vi "create_file_name_discharge (SubVI).vi"(6 "file_idx":i32, 8 "num files":i32, 9 "Electrode settings:":T1={"Electrode to sweep:"=3, "amplitude (V)"=2.0, "frequency (Hz)"=41.0, "offset (V)"=0.0, "Sweep electrode?"=TRUE, "Control DDS"=TRUE}, 10 "base name":string, 11 "base_path":path) -> (2 "output cluster":T2)   [LabVIEW 2022 SP3]
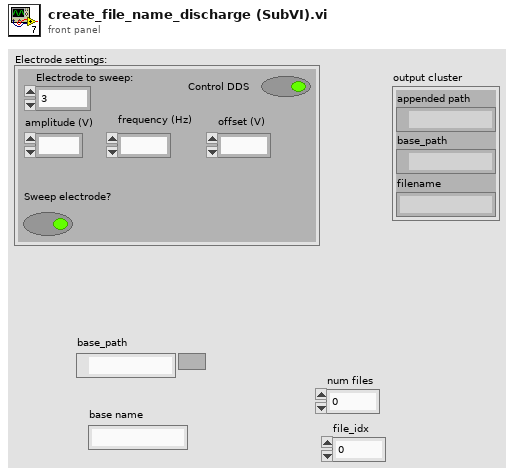
[diagram p1: front panel]
types:
  T1 = cluster{"Electrode to sweep:":i32, "amplitude (V)":ext, "frequency (Hz)":ext, "offset (V)":ext, "Sweep electrode?":bool, "Control DDS":bool}
  T2 = cluster{"appended path":path, "base_path":path, "filename":string}
  T3 = cluster{"appended path":path, "base_path":path, string}
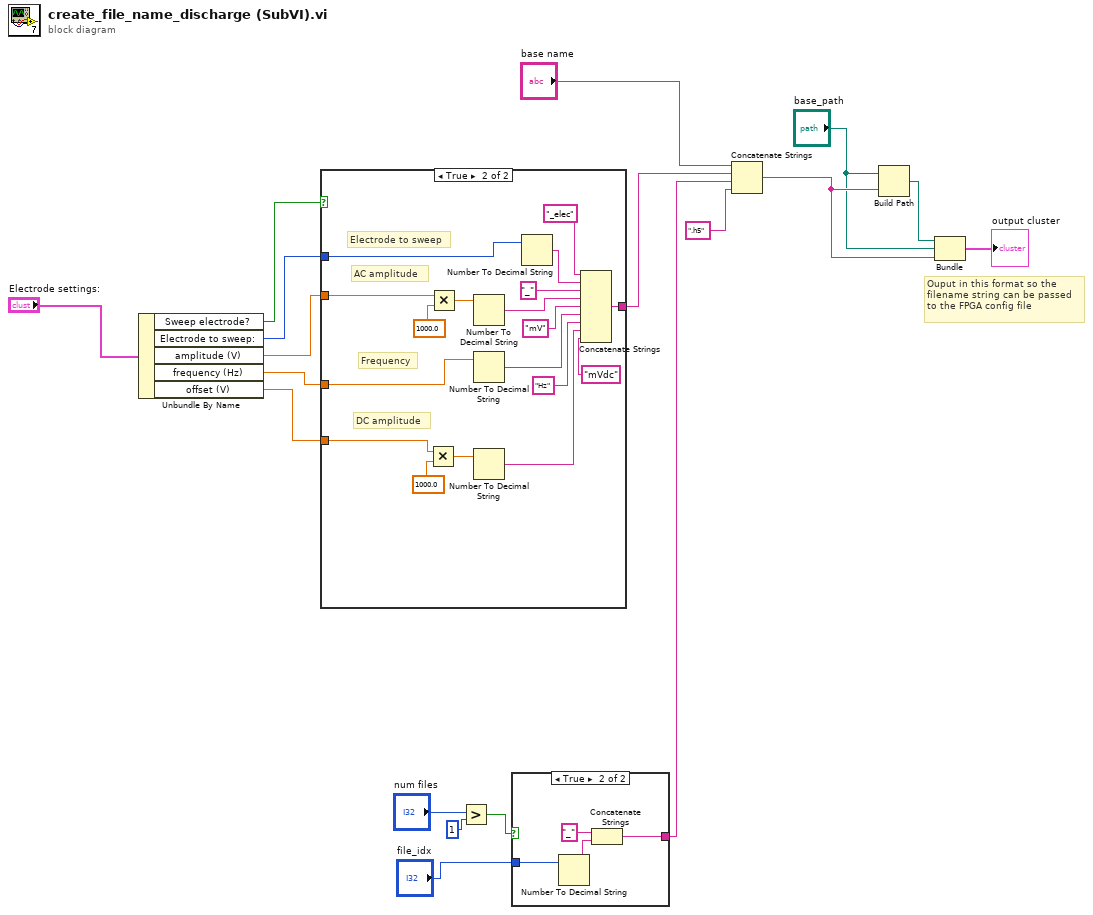
[diagram p0: block diagram]
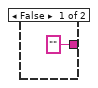
[diagram p2: hidden frame]
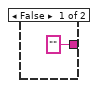
[diagram p3: hidden frame]
diagram:
  # "Ouput in this format so the\nfilename string can be passed\nto the FPGA config file"
  n1 = Unbundle By Name("Electrode settings:") -> ("Sweep electrode?"=w5:bool, "Electrode to sweep:"=w4:i32, "amplitude (V)"=w3:ext, "frequency (Hz)"=w2:ext, "offset (V)"=w1:ext)
  n2 = case shown="True" w5 {
    tunnel: w4 -> [_ w23]
    tunnel: ["" w24] -> w8
    tunnel: w3 -> [_ w22]
    tunnel: w2 -> [_ w21]
    tunnel: w1 -> [_ w20]
    frame False {
    }
    frame True {
      # "DC amplitude"
      # "Frequency"
      # "AC amplitude"
      # "Electrode to sweep"
      n3 = Multiply(x=w20, y=1000.0) -> (x*y=w31:ext)
      n4 = Multiply(x=w22, y=1000.0) -> (x*y=w32:ext)
      n5 = Number To Decimal String(number=w32) -> (decimal integer string=w30:string)  [unwired: 1 in]
      n6 = Number To Decimal String(number=w21) -> (decimal integer string=w28:string)  [unwired: 1 in]
      n7 = Number To Decimal String(number=w31) -> (decimal integer string=w26:string)  [unwired: 1 in]
      n8 = Number To Decimal String(number=w23) -> (decimal integer string=w36:string)  [unwired: 1 in]
      n9 = Concatenate Strings("_elec" ("string"), w36, "_" ("string"), w30, "mV" ("string"), w28, "Hz" ("string"), w26, "mVdc" ("string")) -> (w24:string)
    }
  }
  n10 = Greater?(x="num files", y=1) -> (0:w15:bool)
  n11 = case shown="True" w15 {
    tunnel: "file_idx" -> [_ w41]
    tunnel: ["" w39] -> w7
    frame False {
    }
    frame True {
      n12 = Number To Decimal String(number=w41) -> (decimal integer string=w40:string)  [unwired: 1 in]
      n13 = Concatenate Strings("_" ("string"), w40) -> (w39:string)
    }
  }
  n14 = Concatenate Strings("base name", w8, w7, ".h5" ("string")) -> (w12:string)
  n15 = Build Path(base path="base_path", name or relative path=w12) -> (appended path=w13:path)
  n16 = Bundle("appended path"=w13, "base_path"="base_path", w12) -> (→"output cluster":T3)  [unwired: 1 in]
